vi "Get VI Reference by Name.vi"(8 "error in":errorcluster, 10 "VI name":string, 11 "state in":T1) -> (0 "error out":errorcluster, 1 "found?":bool, 2 "VI ref":refnum<vi>, 3 "state out":T1)   [LabVIEW 2010, in "NI_SE_Config Front Panel Layout.lvlib"]
uses:
  NI_SE_Config Front Panel Layout.lvlib
  State.ctl
  VI Info.ctl
  VI Panel Layout/VI Panel Layout.lvclass
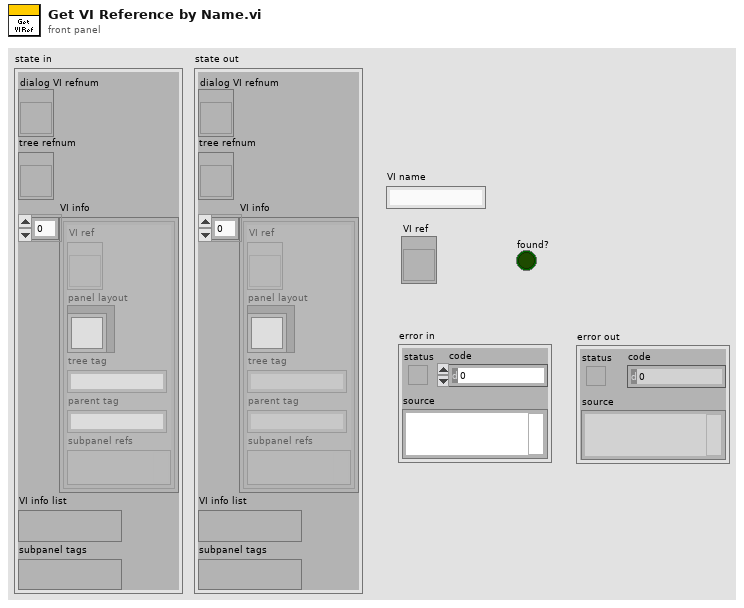
[diagram p1: front panel]
types:
  T1 = typedef "NI_SE_Config Front Panel Layout.lvlib/State.ctl" = cluster{"dialog VI refnum":refnum<vi>, "tree refnum":refnum<vi>, "VI info":T2[], "VI info list":variant, "subpanel tags":variant}
  T2 = typedef "NI_SE_Config Front Panel Layout.lvlib/VI Info.ctl" = cluster{"VI ref":refnum<vi>, "panel layout":refnum<class "VI Panel Layout.lvclass">, "tree tag":string, "parent tag":string, "subpanel refs":variant}
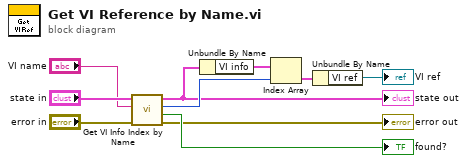
[diagram p0: block diagram]
diagram:
  n1 = call "Get VI Info Index by Name.vi"("error in"="error in", "VI name"="VI name", "state in"="state in") -> ("error out"=→"error out":errorcluster, "found?"=→"found?":bool, "VI info index"=w6:i32, "state out"=w2:T1)  [unwired: 5 in]
  "state out" <- w2
  n2 = Unbundle By Name(w2) -> ("VI info"=w7:T2[])
  n3 = Index Array(array=w7, index=w6) -> (element=w4:T2)
  n4 = Unbundle By Name(w4) -> ("VI ref"=→"VI ref":refnum<vi>)
